vi "Ack Overpressure.vi"(8 "error in (no error)":errorcluster, 11 "ASIA Pump C Settings in":T1) -> (0 "error out":errorcluster)   [LabVIEW 2018, in "ASIA Pump.lvlib"]
uses:
  ASIA Pump.lvlib
  Pump Settings.ctl
  Program Files (x86)/Pfizer/FAST/data/AsiaPumpInterface.dll
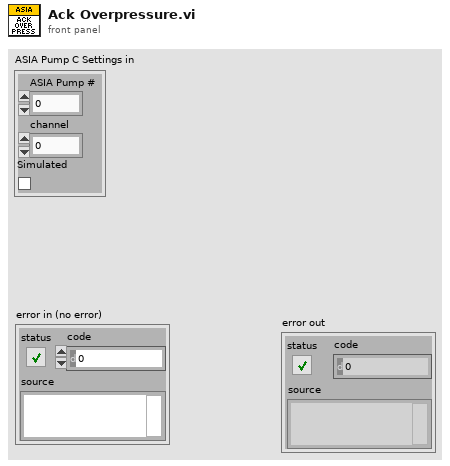
[diagram p1: front panel]
types:
  T1 = typedef "ASIA Pump.lvlib/Pump Settings.ctl" = cluster{"ASIA Pump #":i32, "channel":i32, "Simulated":bool}
  T2 = cluster{"Busy":bool, "PumpCnt":dbl, "RemoteEntered":bool, "OverpressureSet":bool}[]
  T3 = cluster{"Busy":bool, "PumpCnt":dbl, "RemoteEntered":bool, "OverpressureSet":bool}
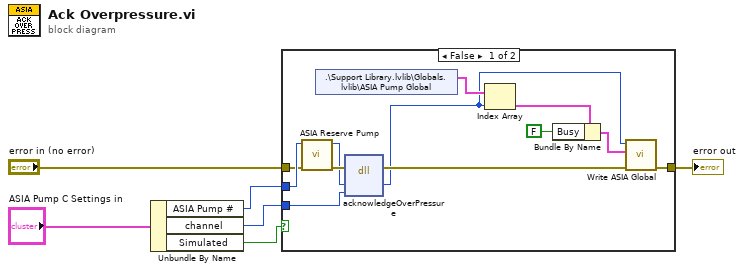
[diagram p0: block diagram]
diagram:
  n1 = Unbundle By Name("ASIA Pump C Settings in") -> ("ASIA Pump #"=w4:i32, "channel"=w2:i32, "Simulated"=w5:bool)
  n2 = case shown="False" w5 {
    tunnel: w4 -> [w18 _]
    tunnel: "error in (no error)" -> [w17 w19]
    tunnel: w2 -> [w10 _]
    tunnel: [w7 w19] -> w1
    frame False {
      n3 = call "ASIA Reserve Pump.vi"("error in (no error)"=w17, "ASIA Pump #"=w18) -> ("error out"=w16:errorcluster, "ASIA Pump #"=w9:i32)  [unwired: 8 in]
      n4 = shared-variable ".\\Support Library.lvlib\\Globals.lvlib\\ASIA Pump Global"() -> (w15:T2)  [unwired: 1 in, 1 out]
      n5 = dll-call lib="C:/Program Files (x86)/Pfizer/FAST/data/AsiaPumpInterface.dll" fn="acknowledgeOverPressure"(error in=w16, "pumpNum"=w9, "channel"=w10) -> (error out=w13:errorcluster, "pumpNum"=w12:u32)  [unwired: 4 in, 1 out]
      n6 = Index Array(array=w15, index=w12) -> (element=w14:T3)
      n7 = Bundle By Name(cluster=w14, "Busy"=FALSE) -> (w11:T3)
      n8 = call "Write ASIA Global.vi"("error in (no error)"=w13, "ASIA Global"=w11, "Pump Number"=w12) -> ("error out"=w7:errorcluster)  [unwired: 7 in, 1 out]
    }
    frame True {
    }
  }
  "error out" <- w1
